vi "错误代码解析.vi"(2 "错误代码":i32) -> (0 "字符串":string, 1 "错误代码":i32)   [LabVIEW 2013]
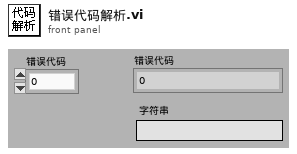
[diagram p1: front panel]
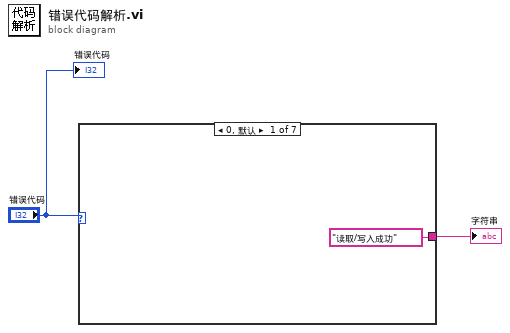
[diagram p0: block diagram]
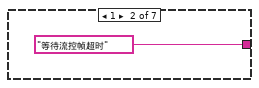
[diagram p2: hidden frame]
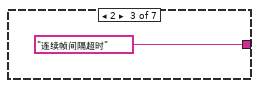
[diagram p3: hidden frame]
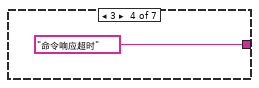
[diagram p4: hidden frame]
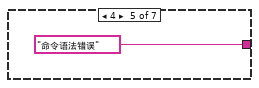
[diagram p5: hidden frame]
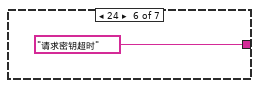
[diagram p6: hidden frame]
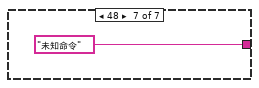
[diagram p7: hidden frame]
diagram:
  n1 = case shown="0, 默认" "错误代码" {
    tunnel: ["读取/写入成功" "等待流控帧超时" "连续帧间隔超时" "命令响应超时" "命令语法错误" "请求密钥超时" "未知命令"] -> w1
    frame 0, Default {
    }
    frame 1 {
    }
    frame 2 {
    }
    frame 3 {
    }
    frame 4 {
    }
    frame 24 {
    }
    frame 48 {
    }
  }
  "字符串" <- w1
  "错误代码" <- "错误代码"
